vi "Write Saved Version.vi"(8 "error in":errorcluster, 10 "Saved Version":string, 11 "PL_System Configuration in":refnum<class "PL_System Configuration.lvclass">) -> (0 "error out":errorcluster, 3 "PL_System Configuration out":refnum<class "PL_System Configuration.lvclass">)   [LabVIEW 2013, in "PL_System Configuration.lvclass"]
uses:
  PL_System Configuration.lvclass
  PL_System Configuration.lvclass/PL_System Configuration.ctl
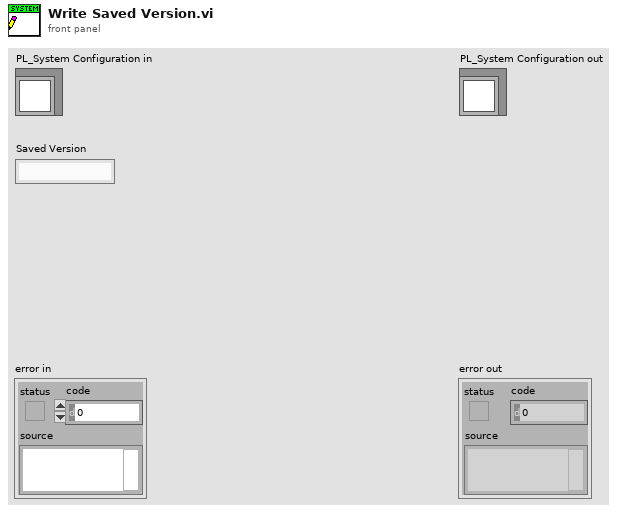
[diagram p1: front panel]
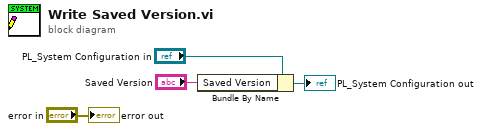
[diagram p0: block diagram]
diagram:
  n1 = Bundle By Name(cluster="PL_System Configuration in", "Saved Version"="Saved Version") -> (→"PL_System Configuration out":refnum<class "PL_System Configuration.lvclass">)
  "error out" <- "error in"
